vi "File Page - Select Waveforms.vi"(8 "error in (no error)":errorcluster, 9 "Item Ref in":T1 format="%.0x", 10 "Events in":string[](array[string]), 11 "File Waveforms in":T2 {"Node Refs" format="%.0x"}) -> (0 "error out":errorcluster, 2 "Events out":string[](array[string]), 3 "File Waveforms out":T2 {"Node Refs" format="%.0x"})   [LabVIEW 2012, in "Waveform Data Logger System Explorer.lvlib"]
uses:
  Waveform Data Logger System Explorer.lvlib
  Types/File - Waveforms.ctl
  <vilib>/NI Veristand/Custom Device API/Custom Device Item Ref.ctl
  Shared/Globals/Global GUIDs.vi
  Shared/Globals/Property Strings.vi
  <userlib>/_OpenG.lib/array/array.llb/Filter 1D Array (U64)__ogtk.vi
  <userlib>/_OpenG.lib/array/array.llb/Reorder 1D Array2 (U32)__ogtk.vi
  <userlib>/_OpenG.lib/array/array.llb/Reorder 1D Array2 (String)__ogtk.vi
  <userlib>/_OpenG.lib/array/array.llb/Reorder 1D Array2 (U64)__ogtk.vi
  <vilib>/NI Veristand/Custom Device API/Set Item Property (String Array).vi
  <vilib>/NI Veristand/Custom Device API/Set Item Property (U32 Array).vi
  <vilib>/NI VeriStand/Custom Device Tools/Custom Device Utility Library/Custom Device Utility Library.lvlib
  <vilib>/NI VeriStand/Custom Device API/Custom Device API.lvlib
  Shared/Waveform Data Logger Shared.lvlib
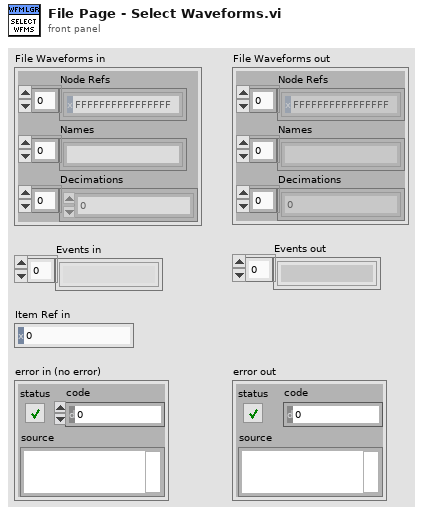
[diagram p1: front panel]
types:
  T1 = typedef "Custom Device API.lvlib/Custom Device Item Ref.ctl" = u64
  T2 = typedef "Waveform Data Logger System Explorer.lvlib/File - Waveforms.ctl" = cluster{"Node Refs":T1[], "Names":string[], "Decimations":u32[]}
  T3 = typedef "Custom Device API.lvlib/Custom Device Item Info.ctl" = cluster{"Name":string, "Is Channel":bool, "GUID":string, "Is Waveform":bool}
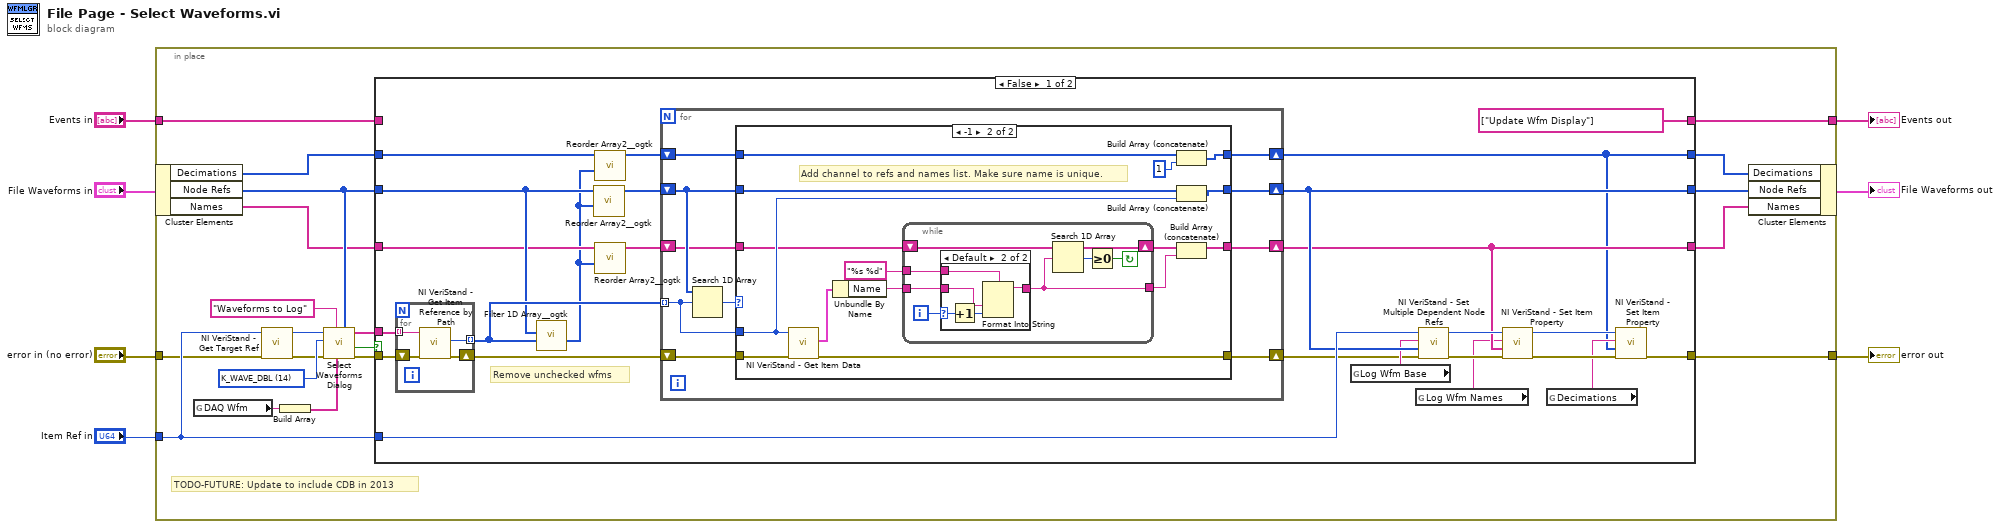
[diagram p0: block diagram]
diagram:
  n1 = in-place {
    in-place-border: "Events in" -> [w27]
    in-place-border: [w26] -> w6
    in-place-border: "Item Ref in" -> [w23]
    in-place-border: [w19] -> w4
    in-place-border: "error in (no error)" -> [w14]
    w17 = u8 14 items=["K_CHAN_R", "K_CHAN_W", "K_CHAN_RW", "K_CHAN_VOLT", "K_CHAN_FAULT", "K_ALL", "K_CUSTOM", "K_CHAN_R_VIS", "K_CHAN_W_VIS", "K_CHAN_RW_VIS", "K_CHAN_VOLT_VIS", "K_CHAN_FAULT_VIS", "K_WAVE", "K_WAVE_VIS", "K_WAVE_DBL", "K_WAVE_CDB", "K_WAVE_DBL_VIS", "K_WAVE_CDB_VIS"] ("Filter")
    # "TODO-FUTURE: Update to include CDB in 2013"
    n2 = in-place-cluster #1("File Waveforms in") -> ("Decimations"=w13:u32[], "Node Refs"=w11:T1[], "Names"=w10:string[])
    n3 = global read "Global GUIDs.vi" "DAQ Wfm"() -> (w24:string)
    n4 = call <vilib>:"NI VeriStand - Get Target Ref.vi"("error in"=w14, "Item Ref in"=w23) -> ("error out"=w15:errorcluster, "Target Ref"=w16:T1)  [unwired: 6 in, 2 out]
    n5 = Build Array(w24) -> (w25:string[])
    n6 = call "Select Waveforms Dialog.vi"("Selected Channel Refs"=w11, "Expand GUIDs"=w25, "Channel Label"="Waveforms to Log", "error in (no error)"=w15, "Filter"=w17, "Start Item Ref"=w16) -> ("error out"=w21:errorcluster, "Canceled"=w22:bool, "Channels"=w20:string[])  [unwired: 3 in]
    n7 = case shown="False" w22 {
      tunnel: w11 -> [w41 w103]
      tunnel: w21 -> [w46 w102]
      tunnel: w20 -> [w45 _]
      tunnel: [w50 w103] -> w9
      tunnel: [w31 w102] -> w26
      tunnel: w23 -> [w51 _]
      tunnel: [string[] ["Update Wfm Display"] w99] -> w19
      tunnel: w10 -> [w39 w101]
      tunnel: [w47 w101] -> w8
      tunnel: w13 -> [w34 w100]
      tunnel: [w30 w100] -> w12
      tunnel: w27 -> [_ w99]
      frame False {
        # "Remove unchecked wfms"
        n8 = for {
          shift-right: [w55] -> w29
          shift-left: w46 -> [w56]
          tunnel: w45 -> [w54] mode=indexing
          tunnel: [w53] -> w42 mode=indexing
          n9 = call <vilib>:"NI VeriStand - Get Item Reference by Path.vi"("error in (no error)"=w56, "Item Path in"=w54) -> ("error out"=w55:errorcluster, "Item Ref"=w53:T1)  [unwired: 6 in, 2 out]
        }
        n10 = call-poly <userlib>:"Filter 1D Array__ogtk.vi"("items to filter"=w42, "array"=w41) -> ("filtered item indices"=w33:i32[])  [unwired: 4 in, 1 out]
        n11 = call-poly <userlib>:"Reorder Array2__ogtk.vi"("indices"=w33, "array"=w41) -> ("reordered array"=w40:u64[])  [unwired: 9 in]
        n12 = call-poly <userlib>:"Reorder Array2__ogtk.vi"("indices"=w33, "array"=w34) -> ("reordered array"=w32:u32[])  [unwired: 9 in]
        n13 = call-poly <userlib>:"Reorder Array2__ogtk.vi"("indices"=w33, "array"=w39) -> ("reordered array"=w38:string[])  [unwired: 9 in]
        n14 = for {
          shift-right: [w64] -> w50
          shift-left: w40 -> [w65]
          shift-right: [w62] -> w47
          shift-left: w38 -> [w63]
          tunnel: w42 -> [w61] mode=indexing
          shift-right: [w59] -> w30
          shift-left: w32 -> [w60]
          shift-right: [w57] -> w28
          shift-left: w29 -> [w58]
          n15 = Search 1D Array(1D array=w65, element=w61) -> (index of element=w66:i32)  [unwired: 1 out]
          n16 = case shown="-1" w66 {
            tunnel: w65 -> [w70 w85]
            tunnel: [w70 w84] -> w64
            tunnel: w61 -> [_ w83]
            tunnel: w63 -> [w69 w78]
            tunnel: [w69 w81] -> w62
            tunnel: w60 -> [w68 w75]
            tunnel: [w68 w73] -> w59
            tunnel: w58 -> [w67 w72]
            tunnel: [w67 w71] -> w57
            frame Default {
              # "Channel already selected for logging. Don't add to refs or names list."
            }
            frame -1 {
              # "Add channel to refs and names list. Make sure name is unique."
              n17 = call <vilib>:"NI VeriStand - Get Item Data.vi"("error in (no error)"=w72, "Item Ref in"=w83) -> ("error out"=w71:errorcluster, "Item Info"=w82:T3)  [unwired: 8 out]
              n18 = Unbundle By Name(w82) -> ("Name"=w77:string)
              n19 = while {
                shift-right: [w90] -> w79
                shift-left: w78 -> [w90]
                tunnel: w77 -> [w91]
                tunnel: [w87] -> w76
                tunnel: "%s %d" ("format string") -> [w86]
                i -> [w92]
                stop <- w88 continue-if-true
                n20 = case shown="Default" w92 {
                  selector: w92 -> [_ w96]
                  tunnel: w91 -> [w93 w94]
                  tunnel: [w93 w98] -> w87
                  tunnel: w86 -> [_ w97]
                  frame 0 {
                  }
                  frame Default {
                    n21 = Increment(x=w96) -> (x+1=w95:i32)
                    n22 = Format Into String(format string=w97, w94, w95) -> (resulting string=w98:string)  [unwired: 2 in, 1 out]
                  }
                }
                n23 = Search 1D Array(1D array=w90, element=w87) -> (index of element=w89:i32)  [unwired: 1 out]
                n24 = Greater Or Equal To 0?(x=w89) -> (x >= 0?=w88:bool)
              }
              n25 = Build Array (concatenate)(w75, u32 1) -> (w73:u32[])
              n26 = Build Array (concatenate)(w85, w83) -> (w84:T1[])
              n27 = Build Array (concatenate)(w79, w76) -> (w81:string[])
            }
          }
        }
        n28 = global read "Property Strings.vi" "Log Wfm Base"() -> (w44:string)
        n29 = global read "Property Strings.vi" "Log Wfm Names"() -> (w43:string)
        n30 = call <vilib>:"NI VeriStand - Set Multiple Dependent Node Refs.vi"("error in (no error)"=w28, "Dependent Node Refs"=w50, "Base Property Name"=w44, "Item Ref in"=w51) -> ("error out"=w48:errorcluster, "Item Ref out"=w49:T1)  [unwired: 6 in]
        n31 = call-poly <vilib>:"NI VeriStand - Set Item Property.vi"("error in (no error)"=w48, "Value"=w47, "Property Name"=w43, "Item Ref in"=w49) -> ("error out"=w36:errorcluster, "Item Ref out"=w37:T1)  [unwired: 5 in, 1 out]
        n32 = global read "Property Strings.vi" "Decimations"() -> (w35:string)
        n33 = call-poly <vilib>:"NI VeriStand - Set Item Property.vi"("error in (no error)"=w36, "Value"=w30, "Property Name"=w35, "Item Ref in"=w37) -> ("error out"=w31:errorcluster)  [unwired: 5 in, 2 out]
      }
      frame True {
        # "User canceled out of the dialog."
      }
    }
    n34 = in-place-cluster #1("Decimations"=w12, "Node Refs"=w9, "Names"=w8) -> (→"File Waveforms out":T2)
  }
  "error out" <- w6
  "Events out" <- w4
